vi "RSZVB Set IMOD Upper Tone Source.vi"(7 "Source Number (1)":i32=1, 8 "error in (no error)":errorcluster {"code" format="%.0x"}, 9 "Source (0: Port)":i32(ring) items=["Port", "Generator"], 10 "Channel (1)":i32=1, 11 "VISA session":refnum<visa-resource-name>) -> (0 "error out":errorcluster {"code" format="%.0x"}, 3 "dup VISA session":refnum<visa-resource-name>)   [LabVIEW 2011]
doc: "This VI selects the source for the upper tone signal that is used for the intermodulation measurement.\n\nNote(s):\n\n(1) This VI is not available for R&S ZVB instrument.\n\nRemote-control command(s):\n[SENSe<Ch>:]FREQuency:IMODulation:UTONe NONE | PORT | GENerator, <source_no>"
uses:
  _utility/RSZVB Global Data.vi
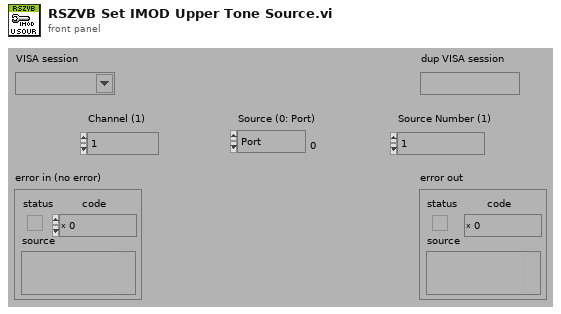
[diagram p1: front panel]
types:
  T1 = cluster{"Error Checking (T: On)":bool, "Installed Options":string[], "Data Valid?":bool, "Ports":i32, "Model":string[], "Option Checking (T: On)":bool}[]
  T2 = cluster{"Error Checking (T: On)":bool, "Installed Options":string[], "Data Valid?":bool, "Ports":i32, "Model":string[], "Option Checking (T: On)":bool}
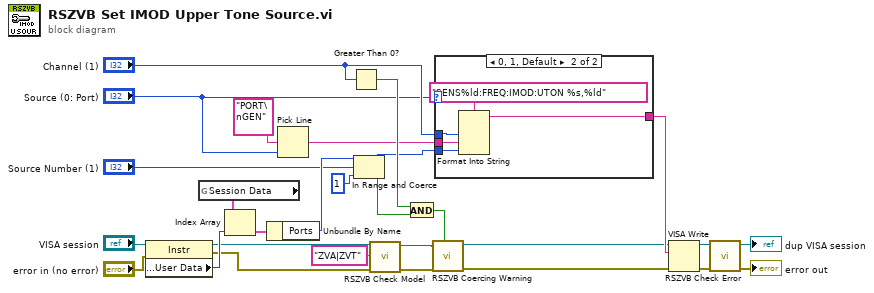
[diagram p0: block diagram]
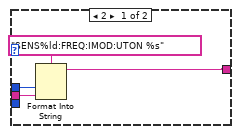
[diagram p2: hidden frame]
diagram:
  n1 = property class="Instr"(reference="VISA session", error in="error in (no error)") -> (reference out=w2:refnum<visa-resource-name>, error out=w3:errorcluster, "General Settings:User Data"=w13:u32)
  n2 = global read "RSZVB Global Data.vi" "Session Data"() -> (w14:T1)
  n3 = Index Array(array=w14, index=w13) -> (element=w15:T2)
  n4 = Unbundle By Name(w15) -> ("Ports"=w22:i32)
  n5 = Pick Line(multi-line string="PORT\nGEN", line index="Source (0: Port)") -> (output string=w21:string)  [unwired: 1 in]
  n6 = Greater Than 0?(x="Channel (1)") -> (x > 0?=w26:bool)
  n7 = In Range and Coerce(upper limit=w22, x="Source Number (1)", lower limit=1) -> (coerced(x)=w24:i32, In Range?=w25:bool)
  n8 = call "RSZVB Check Model.vi"("error in (no error)"=w3, "Model"="ZVA|ZVT", "VISA session"=w2) -> ("error out"=w4:errorcluster, "dup VISA session"=w5:refnum<visa-resource-name>)  [unwired: 7 in]
  n9 = And(x=w26, y=w25) -> (x .and. y?=w27:bool)
  n10 = call "RSZVB Coercing Warning.vi"("In Range?"=w27, "error in (no error)"=w4, "VISA session"=w5) -> ("error out"=w18:errorcluster, "dup VISA session"=w19:refnum<visa-resource-name>)  [unwired: 7 in]
  n11 = case shown="0, 1, Default" "Source (0: Port)" {
    tunnel: w21 -> [w31 w36]
    tunnel: w24 -> [_ w35]
    tunnel: [w30 w34] -> w28
    tunnel: "Channel (1)" -> [w29 w33]
    frame 2 {
      n12 = Format Into String(format string="SENS%ld:FREQ:IMOD:UTON %s", w29, w31) -> (resulting string=w30:string)  [unwired: 2 in, 1 out]
    }
    frame 0, 1, Default {
      n13 = Format Into String(format string="SENS%ld:FREQ:IMOD:UTON %s,%ld", w33, w36, w35) -> (resulting string=w34:string)  [unwired: 2 in, 1 out]
    }
  }
  n14 = VISA Write(VISA resource name=w19, write buffer=w28, error in (no error)=w18) -> (VISA resource name out=w16:refnum<visa-resource-name>, error out=w17:errorcluster)  [unwired: 1 out]
  n15 = call "RSZVB Check Error.vi"("error in (no error)"=w17, "VISA session"=w16) -> ("error out"=→"error out":errorcluster, "dup VISA session"=→"dup VISA session":refnum<visa-resource-name>)  [unwired: 8 in]
